vi "Exercice 3.vi"() -> ()   [LabVIEW 2018]
panel:
  out "LED":bool
  out "Nom":string
  out "Prénom":string
  in  "Nom brut":string
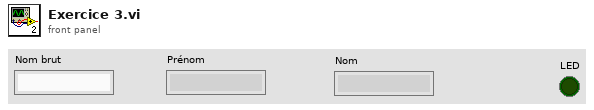
[diagram p1: front panel]
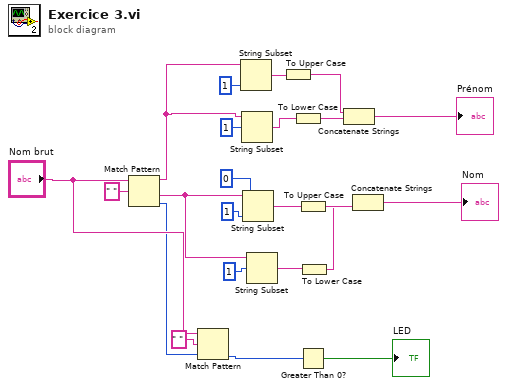
[diagram p0: block diagram]
diagram:
  n1 = Match Pattern(string="Nom brut", regular expression=" ") -> (before substring=w7:string, after substring=w6:string, offset past match=w3:i32)  [unwired: 1 in, 1 out]
  n2 = Match Pattern(string="Nom brut", regular expression=" ", offset (0)=w3) -> (offset past match=w2:i32)  [unwired: 3 out]
  n3 = String Subset(string=w7, length (rest)=1 ("length (rest)")) -> (substring=w22:string)  [unwired: 1 in]
  n4 = String Subset(string=w7, offset (0)=1) -> (substring=w19:string)  [unwired: 1 in]
  n5 = String Subset(string=w6, offset (0)=0, length (rest)=1 ("length (rest)")) -> (substring=w14:string)
  n6 = String Subset(string=w6, offset (0)=1) -> (substring=w11:string)  [unwired: 1 in]
  n7 = To Upper Case(1:w22) -> (0:w21:string)
  n8 = To Lower Case(string=w19) -> (all lower case string=w18:string)
  n9 = To Upper Case(1:w14) -> (0:w15:string)
  n10 = Greater Than 0?(x=w2) -> (x > 0?=→"LED":bool)
  n11 = To Lower Case(string=w11) -> (all lower case string=w10:string)
  n12 = Concatenate Strings(w21, w18) -> (→"Prénom":string)
  n13 = Concatenate Strings(w15, w10) -> (→"Nom":string)
